vi "libssh2_agent_publickey_refnum_create.vi"(8 "error in (no error)":errorcluster, 11 "libssh2_agent_publickey*":u64 format="%.0x") -> (0 "error out":errorcluster, 3 "public key":T1)   [LabVIEW 2013, in "libssh2.lvlib"]
doc: "Creates a <B>public key</B> refnum from a pointer to libssh2_agent_publickey."
uses:
  libssh2.lvlib
  libssh2_agent_publickey_refnum.ctl
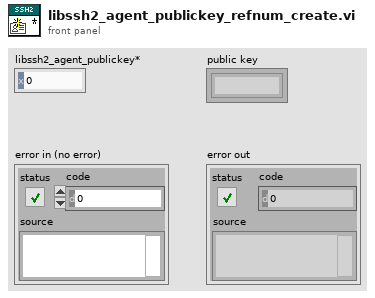
[diagram p1: front panel]
types:
  T1 = typedef "libssh2.lvlib/libssh2_agent_publickey_refnum.ctl" = refnum<k1>
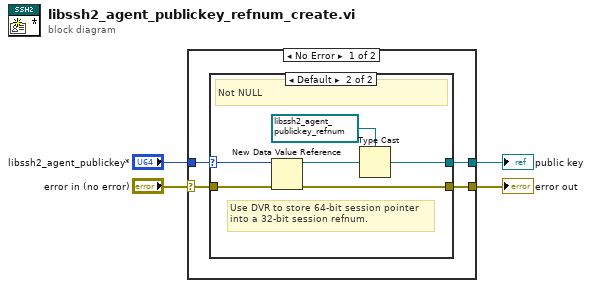
[diagram p0: block diagram]
diagram:
  n1 = case shown="No Error" "error in (no error)" {
    selector: "error in (no error)" -> [w6 w16]
    tunnel: [w8 _] -> w4
    tunnel: [w7 w16] -> w3
    tunnel: "libssh2_agent_publickey*" -> [w5 _]
    frame No Error {
      n2 = case shown="Default" w5 {
        selector: w5 -> [_ w13]
        tunnel: [_ w14] -> w8
        tunnel: [w9 w11] -> w7
        tunnel: w6 -> [w9 w10]
        frame 0 {
          # "NULL"
        }
        frame Default {
          w15 = T1 refnum items=["publickey"] ("libssh2_agent_publickey_refnum")
          # "Use DVR to store 64-bit session pointer\ninto a 32-bit session refnum."
          # "Not NULL"
          n3 = New Data Value Reference(data value=w13, error in=w10) -> (data value reference=w12:refnum<data-value>, error out=w11:errorcluster)
          n4 = Type Cast(type=w15, x=w12) -> (*(type *) &x=w14:T1)
        }
      }
    }
    frame Error {
    }
  }
  "public key" <- w4
  "error out" <- w3
